vi "pb_stop_programming.vi"(8 "error in (no error)":errorcluster, 11 "path in":path=path "C:/Program Files/SpinCore/SpinAPI/dll/spinapi.dll") -> (0 "error out":errorcluster, 3 "path out":path)   [LabVIEW 2013, in "SpinAPI-20140801.lvlib"]
uses:
  SpinAPI-20140801.lvlib
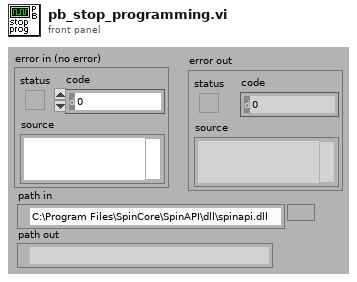
[diagram p1: front panel]
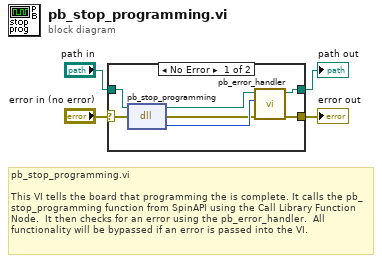
[diagram p0: block diagram]
diagram:
  # "pb_stop_programming.vi\n\nThis VI tells the board that programming the is complete. It calls the pb_stop_programming function from SpinAPI using the Call Library Function Node.  It then checks for an error using the pb_error_handler.  All functionality will be bypassed if an error is passed into the VI."
  n1 = case shown="No Error" "error in (no error)" {
    selector: "error in (no error)" -> [w11 w13]
    tunnel: [w5 w13] -> w3
    tunnel: "path in" -> [w9 w12]
    tunnel: [w6 w12] -> w1
    frame No Error {
      n2 = dll-call lib="C:/Program Files/SpinCore/SpinAPI/dll/spinapi.dll" fn="pb_stop_programming"(path in=w9, error in=w11) -> (path out=w8:path, error out=w7:errorcluster, "return type"=w10:i32)  [unwired: 1 in]
      n3 = call "pb_error_handler.vi"("error in (no error)"=w7, "return code"=w10, "path in"=w8) -> ("error out"=w5:errorcluster, "path out"=w6:path)  [unwired: 7 out]
    }
    frame Error {
    }
  }
  "error out" <- w3
  "path out" <- w1
